vi "Start TDSM.vi"(8 "error in (no error)":errorcluster, 11 "UDP Reader in":refnum<class "UDP Reader.lvclass">) -> (0 "error out":errorcluster, 3 "UDP Reader out":refnum<class "UDP Reader.lvclass">)   [LabVIEW 2022 SP3, in "UDP Reader.lvlib" / "UDP Reader.lvclass"]
uses:
  UDP Reader.lvclass
  C:/Program Files (x86)/National Instruments/LabVIEW 2022/vi.lib/ActorFramework/Actor/Actor.lvclass
  UDP Reader Messages/Read Msg/Read Msg.lvclass
  C:/Program Files (x86)/National Instruments/LabVIEW 2022/vi.lib/ActorFramework/Message/Message.lvclass
  <vilib>/ActorFramework/Message Enqueuer/Message Priority.ctl
  UDP Reader Messages/Feedback Msg/Feedback Msg.lvclass
  <vilib>/ActorFramework/Actor/Actor.lvclass/Actor.ctl
  <vilib>/ActorFramework/Message Enqueuer/Message Enqueuer.lvclass/Message Enqueuer.ctl
  UDP Reader.lvclass/UDP Reader.ctl
  <vilib>/ActorFramework/Message Enqueuer/Init from Existing Queue.vi
  <vilib>/ActorFramework/Message Enqueuer/Message Enqueuer.lvclass
  <vilib>/ActorFramework/Actor/Actor.lvclass
  C:/Users/ebert/Documents/codes/SSL/repo/Phoenix Reborn/UDP Reader/UDP Reader Messages/Read Msg/Read Msg.lvclass
  C:/Program Files (x86)/National Instruments/LabVIEW 2022/vi.lib/MGI/Monitored Actor/Monitored Actor/Monitored Actor/Monitored Actor.lvclass
  C:/Users/ebert/Documents/codes/SSL/repo/Phoenix Reborn/UDP Reader/UDP Reader/UDP Reader.lvclass
  C:/Users/ebert/Documents/codes/SSL/repo/Phoenix Reborn/UDP Reader/UDP Reader Messages/Feedback Msg/Feedback Msg.lvclass
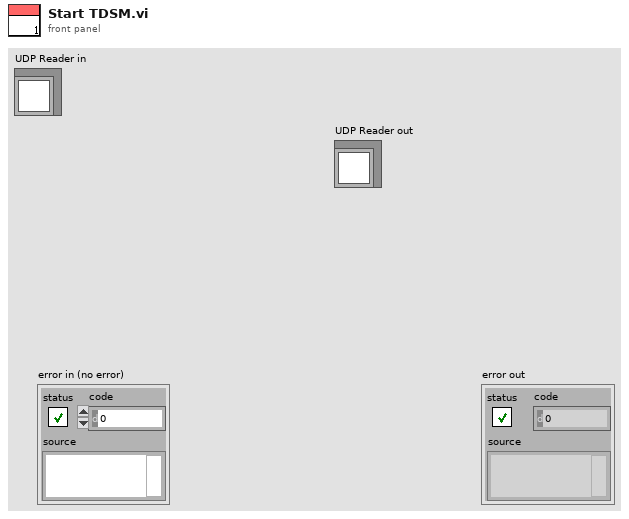
[diagram p1: front panel]
types:
  T1 = typedef "Actor Framework.lvlib/Message Enqueuer.lvclass/Message Priority.ctl" = enum16{"Low", "Normal", "High"}
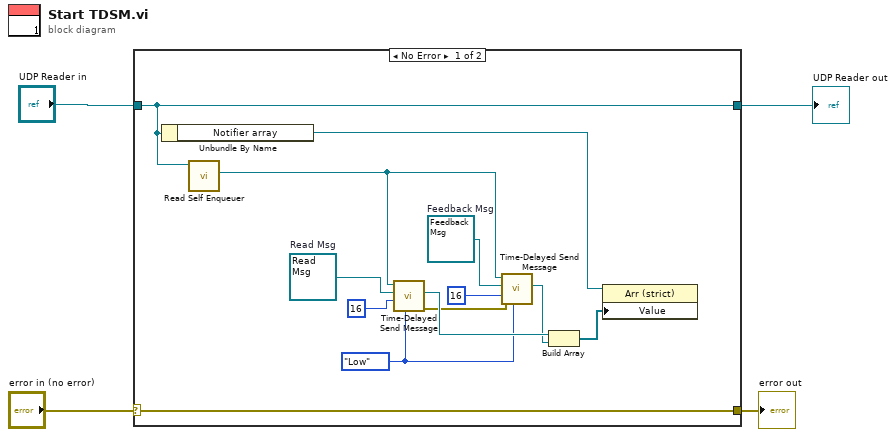
[diagram p0: block diagram]
diagram:
  n1 = case shown="No Error" "error in (no error)" {
    selector: "error in (no error)" -> [w17 w19]
    tunnel: [w17 w19] -> w3
    tunnel: "UDP Reader in" -> [w7 w18]
    tunnel: [w7 w18] -> w1
    frame No Error {
      w5 = refnum<class "Feedback Msg.lvclass"> refnum  # Feedback Msg
      w11 = Message_Priority."Low" ("Message Priority (Normal)")
      w13 = refnum<class "Read Msg.lvclass"> refnum  # Read Msg
      n2 = Unbundle By Name(w7) -> ("Notifier array"=w10:refnum<vi>)
      n3 = call <vilib>:"Read Self Enqueuer.vi"("Actor"=w7) -> ("Self Enqueuer"=w8:refnum<class "Message Enqueuer.lvclass">)  [unwired: 10 in]
      n4 = call <vilib>:"Time-Delayed Send Message.vi"("Message Priority (Normal)"=w11, "Milliseconds To Wait"=16, "Message"=w13, "Message Enqueuer"=w8) -> ("error out"=w15:errorcluster, "Delivery Notifier"=w16:refnum<notifier>)  [unwired: 6 in]
      n5 = call <vilib>:"Time-Delayed Send Message.vi"("Message Priority (Normal)"=w11, "error in (no error)"=w15, "Milliseconds To Wait"=16, "Message"=w5, "Message Enqueuer"=w8) -> ("Delivery Notifier"=w12:refnum<notifier>)  [unwired: 5 in, 1 out]
      n6 = Build Array(w16, w12) -> (w9:refnum<notifier>[])
      n7 = property class="Arr (strict)"(reference=w10, "Value"=w9) -> ()  [unwired: 1 in, 2 out]
    }
    frame Error {
    }
  }
  "error out" <- w3
  "UDP Reader out" <- w1
